vi "Setup.vi"(11 "error in (no error)":errorcluster) -> (4 "Application Ref":refnum<vi>, 6 "VI out":refnum<vi>, 15 "error out":errorcluster)   [LabVIEW 2016, in "DronaTest.lvlib"]
uses:
  DronaTest.lvlib
  Drona.lvlib
  APIs/Assert/AssertVI/Exec/AssertVIExecRunning.vi
  APIs/Assert/AssertVI/AssertVI.lvlib
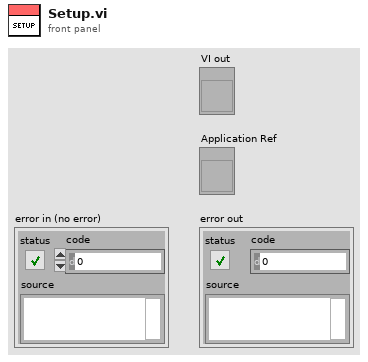
[diagram p1: front panel]
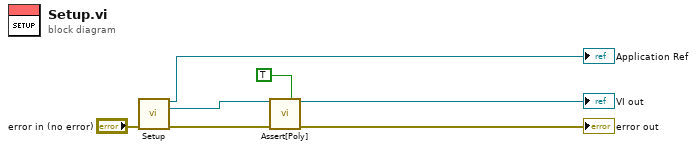
[diagram p0: block diagram]
diagram:
  n1 = call "Setup.vi"("error in"="error in (no error)") -> ("Application Ref"=→"Application Ref":refnum<vi>, "VI Reference Out"=w5:refnum<vi>, "error out"=w3:errorcluster)  [unwired: 12 in]
  n2 = call-poly "Assert[Poly].vi"("VI Reference In"=w5, "Assert Only? (F)"=TRUE, "Error In"=w3) -> ("VI Reference Out"=→"VI out":refnum<vi>, "Error Out"=→"error out":errorcluster)  [unwired: 10 in, 1 out]
